vi "Configure SMU Bandwidth Oscillation.vi"(7 "Enable Oscillation (False)":bool, 8 "error in (no error)":errorcluster {"code" format="%.0x"}, 9 "Voltage Bandwidth (0: Low)":i32(ring) items=["Low", "High1", "High2", "High3"], 10 "Channel Name (1)":string="1", 11 "VISA resource name":refnum<visa-resource-name>) -> (0 "error out":errorcluster {"code" format="%.0x"}, 3 "VISA resource name out":refnum<visa-resource-name>)   [LabVIEW 2018, in "Agilent N6700 Series.lvlib"]
doc: "Sets the voltage bandwidth and oscillation state.\n\n<b>Note:</b>\nThis VI only applies to model N678xA SMU."
uses:
  Agilent N6700 Series.lvlib
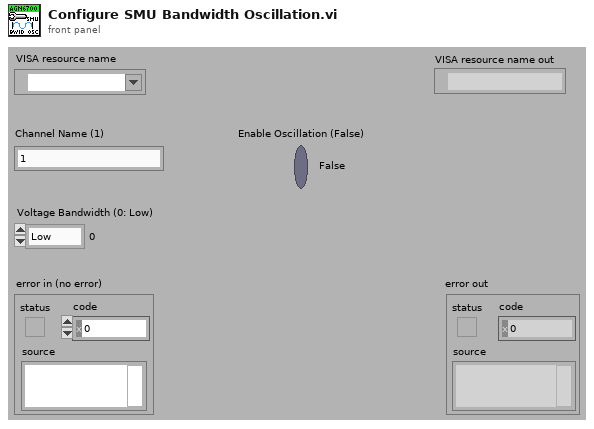
[diagram p1: front panel]
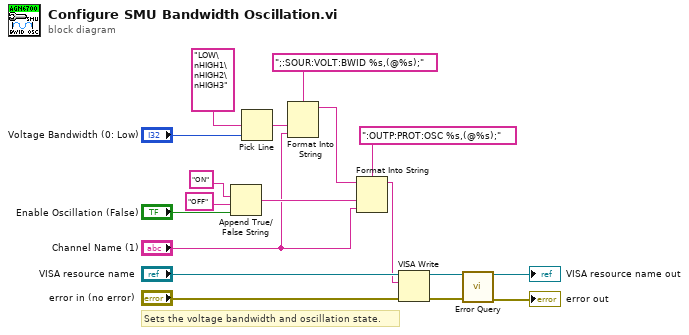
[diagram p0: block diagram]
diagram:
  # "Sets the voltage bandwidth and oscillation state."
  n1 = Append True/False String(1:"Enable Oscillation (False)", 2:"OFF", 3:"ON") -> (0:w3:string)  [unwired: 1 in]
  n2 = Pick Line(multi-line string="LOW\nHIGH1\nHIGH2\nHIGH3" ("string (\"\")"), line index="Voltage Bandwidth (0: Low)") -> (output string=w4:string)  [unwired: 1 in]
  n3 = Format Into String(format string=";:SOUR:VOLT:BWID %s,(@%s);", w4, "Channel Name (1)") -> (resulting string=w12:string)  [unwired: 2 in, 1 out]
  n4 = Format Into String(format string=":OUTP:PROT:OSC %s,(@%s);", initial string=w12, w3, "Channel Name (1)") -> (resulting string=w7:string)  [unwired: 1 in, 1 out]
  n5 = VISA Write(VISA resource name="VISA resource name", write buffer=w7, error in (no error)="error in (no error)") -> (VISA resource name out=w14:refnum<visa-resource-name>, error out=w13:errorcluster)  [unwired: 1 out]
  n6 = call "Error Query.vi"("VISA resource name"=w14, "error in (no error)"=w13) -> ("VISA resource name out"=→"VISA resource name out":refnum<visa-resource-name>, "error out"=→"error out":errorcluster)  [unwired: 10 in, 2 out]
